vi "Funcion_Escribir.vi"() -> ()   [LabVIEW 2016]
uses:
  microchip_solutions_v2013-06-15/USB/Tools/MCHPUSB Custom Driver/Mpusbapi/Dll/Borland_C/mpusbapi.dll
panel:
  out "pLength":i32
  in  "PIPE OUT":i32
  out "string":string
  out "number":u32
  in  "Array":bool[](array[boolean])
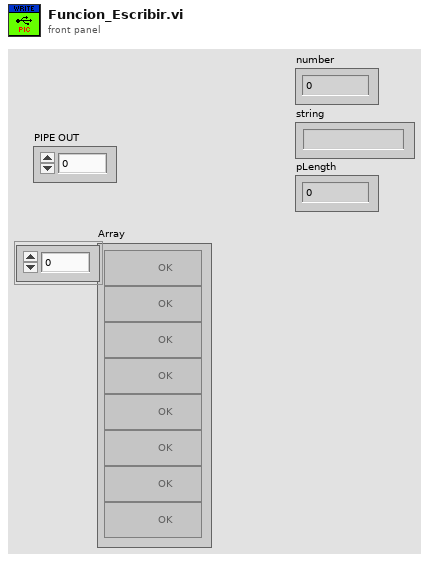
[diagram p1: front panel]
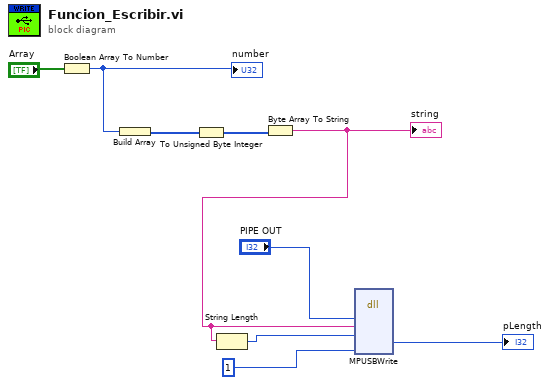
[diagram p0: block diagram]
diagram:
  n1 = Boolean Array To Number(Boolean array="Array") -> (number=w7:u32)
  "number" <- w7
  n2 = Build Array "Build Array"(w7) -> (w8:u32[])
  n3 = To Unsigned Byte Integer(number=w8) -> (unsigned 8bit integer=w6:u8[])
  n4 = Byte Array To String(unsigned byte array=w6) -> (string=w4:string)
  "string" <- w4
  n5 = String Length(string=w4) -> (length=w3:i32)
  n6 = dll-call lib="C:/microchip_solutions_v2013-06-15/USB/Tools/MCHPUSB Custom Driver/Mpusbapi/Dll/Borland_C/mpusbapi.dll" fn="MPUSBWrite"("PIPE OUT"="PIPE OUT", "pData"=w4, "dwLength"=w3, "Milliseconds"=1) -> ("pLength"=→"pLength":i32)  [unwired: 9 in, 2 out]
